vi "send_receive_p.vi"() -> ()   [LabVIEW 2010]
uses:
  <userlib>/libcommon_serial/libcommon_serial.lvlib
panel:
  out "serial_handle":u32
  out "Timeout Reading":bool
  out "Timeout Writing":bool
  out "Byte received":i32[](array[numeric])
  out "Byte Sent":i32[](array[numeric])
  out "Error testing ramp":bool
  out "Not read all bytes":bool
  out "Not written all bytes":bool
  in  "timeo":i32
  in  "Test Buffer size":i32=128
  in  "bits":i32=8
  in  "stop":i32=1
  in  "parity":i32
  in  "baudrate":i32=115200
  in  "serdev":string="/dev/ttyr00"
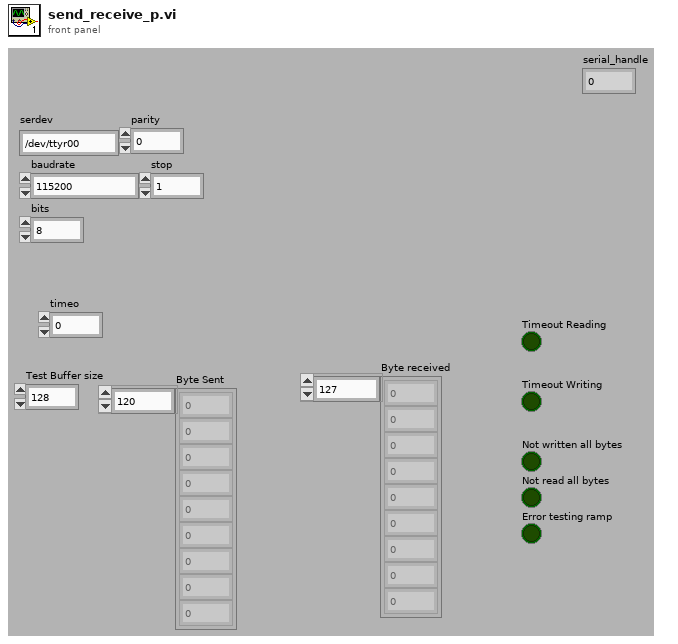
[diagram p1: front panel]
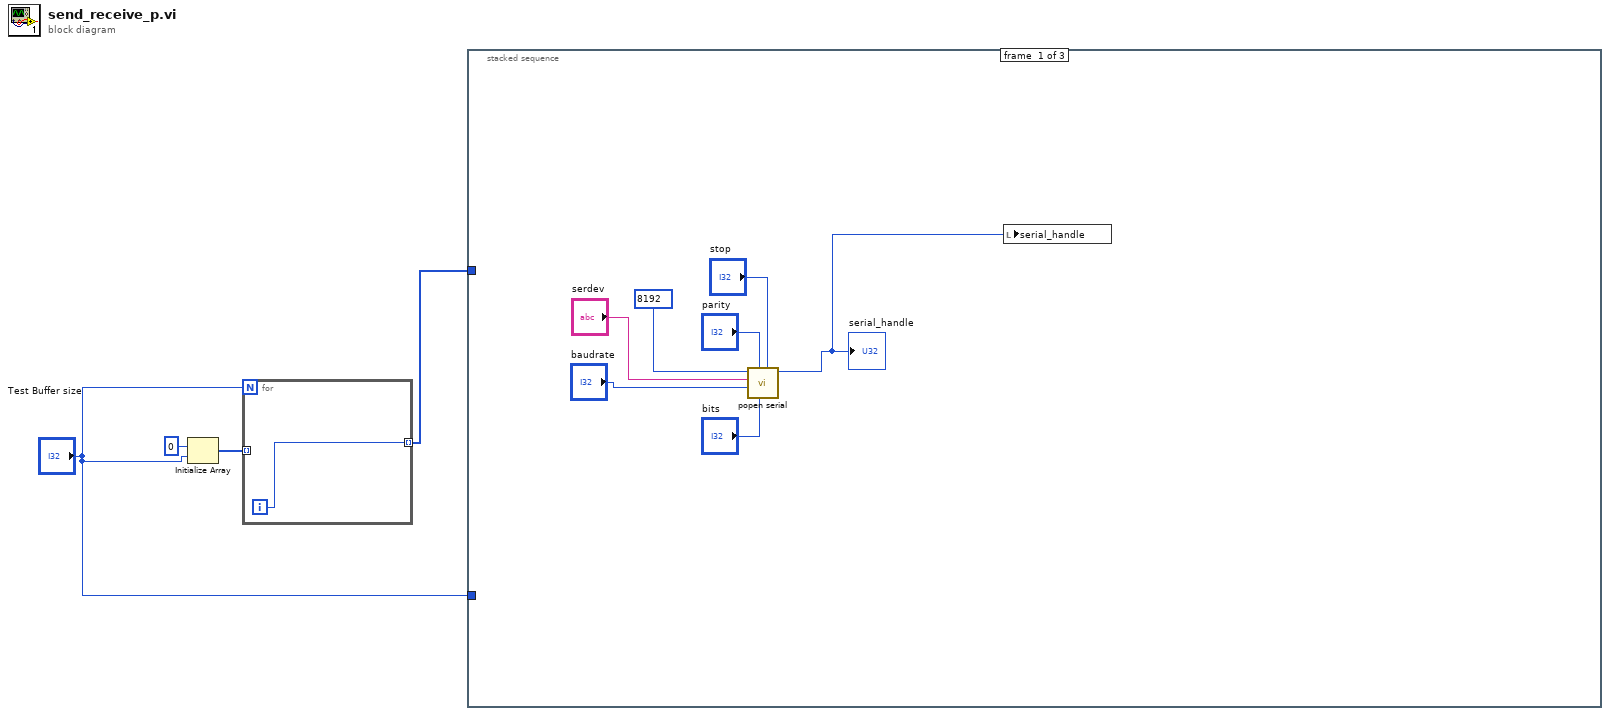
[diagram p0: block diagram]
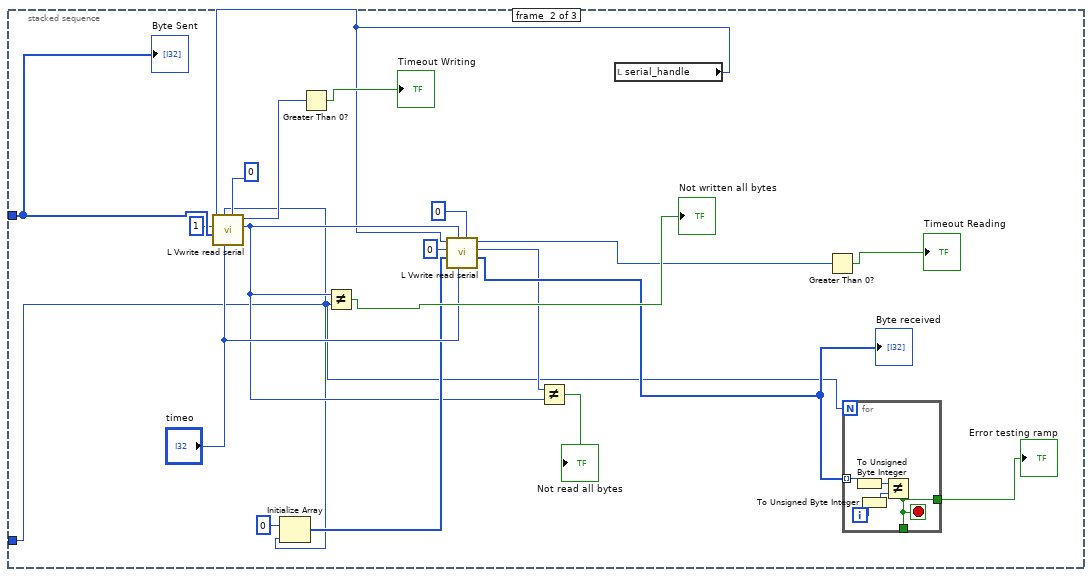
[diagram p2: hidden frame]
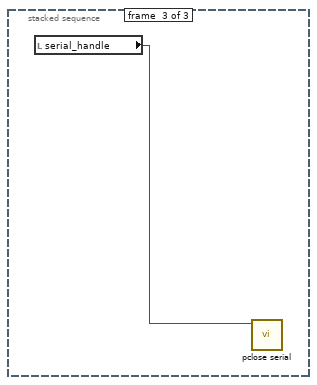
[diagram p3: hidden frame]
diagram:
  n1 = Initialize Array(i8 0 ("element"), "Test Buffer size") -> (w3:i8[])
  n2 = for {
    N: "Test Buffer size" -> [_]
    tunnel: w3 -> [_] mode=indexing
    tunnel: [w5] -> w2 mode=indexing
    i -> [w5]
  }
  n3 = stacked-sequence {
    tunnel: w2 -> [_ w27 _]
    tunnel: "Test Buffer size" -> [_ w14 _]
    frame #0 {
      n4 = call <userlib>:"popen serial.vi"("stop"="stop", "bits"="bits", "parity"="parity", "baudrate"="baudrate", "serdev"="serdev", "internal_buffering"=8192) -> ("serial_handle"=w6:u32)  [unwired: 4 in, 1 out]
      "serial_handle" <- w6
      n5 = local write "serial_handle"(w6) -> ()
    }
    frame #1 {
      n6 = Initialize Array(i8 0 ("element"), w14) -> (w24:i8[])
      n7 = local read "serial_handle"() -> (w13:u32)
      n8 = call <userlib>:"L Vwrite read serial.vi"("timoccur"=0, "timeo"="timeo", "bsize"=w14, "buf"=w27, "iswrite"=1, "h"=w13) -> ("bytes w/r"=w17:i32, "timoccur out"=w32:i32)  [unwired: 3 in, 1 out]
      n9 = Greater Than 0?(x=w32) -> (x > 0?=→"Timeout Writing":bool)
      n10 = Not Equal?(x=w17, y=w14) -> (x != y?=→"Not written all bytes":bool)
      n11 = call <userlib>:"L Vwrite read serial.vi"("timoccur"=0, "timeo"="timeo", "bsize"=w17, "buf"=w24, "iswrite"=0, "h"=w13) -> ("buf out"=w22:i8[], "bytes w/r"=w16:i32, "timoccur out"=w23:i32)  [unwired: 3 in]
      "Byte received" <- w22
      n12 = Not Equal?(x=w16, y=w17) -> (x != y?=→"Not read all bytes":bool)
      n13 = Greater Than 0?(x=w23) -> (x > 0?=→"Timeout Reading":bool)
      n14 = for {
        N: w14 -> [_]
        tunnel: w22 -> [w36] mode=indexing
        tunnel: [w33] -> _
        tunnel: [w33] -> w28
        i -> [w37]
        stop <- w33 stop-if-true
        n15 = To Unsigned Byte Integer(number=w36) -> (unsigned 8bit integer=w35:u8)
        n16 = To Unsigned Byte Integer(number=w37) -> (unsigned 8bit integer=w34:u8)
        n17 = Not Equal?(x=w35, y=w34) -> (x != y?=w33:bool)
      }
      "Error testing ramp" <- w28
      "Byte Sent" <- w27
    }
    frame #2 {
      n18 = local read "serial_handle"() -> (w38:u32)
      n19 = call <userlib>:"pclose serial.vi"("h"=w38) -> ()  [unwired: 10 in, 1 out]
    }
  }
